vi "DriverStationSendData.vi"   [LabVIEW 2020]
doc: "This VI continously sends data from the robot to the FRC 4265 Dashboard, the joysticks, and the FIRST Driver Station. Data are only sent to the network tables when values change. Detailed sensor data are only sent when the user is currently viewing the Tune tab on the FRC 4265 Dashboard."
uses:
  <vilib>/Rock Robotics/WPI/DriverStation/WPI_DriverStationAllianceInfo.ctl
  0776bb0e-5b58-4af6-957d-bc8a00d122f2.vi
  c0b3d222-824d-4eea-b194-4551ccfede72.vi
  fb3b5982-3a93-47f1-af4b-9be2dbb142fb.vi
  9698e8dd-c256-4803-872d-8995bd52a814.vi
  549dd589-3d40-49fe-b500-ea8f2f2c089b.vi
  770be32f-1451-480f-be59-c95d907125ff.vi
  66123533-5387-4bde-a965-6a0533df74da.vi
  63beb643-7217-41a5-919e-8b0b42428238.vi
  f953088c-0ff5-4157-aadb-ae5236f80662.vi
  9b798e4d-9237-4864-9935-e997a6382231.vi
  bf36f1cc-a3b1-4189-9382-aff2debcdd91.vi
  09cab74e-98ba-4de8-92cd-b77291f0cae9.vi
  e0f98f21-d526-4ef5-b75c-6f3c78a33603.vi
  ae67384e-06ed-4288-bfa6-012d261b0193.vi
  36759aca-d9c6-44a3-918a-9a0e895c718f.vi
  d2dc3f3f-39b5-4c17-a933-05bbedc8d5d9.vi
  47e8091e-0604-4560-b6ee-932fcc40f94c.vi
  040c557e-2b24-4d13-8fef-d98c711cf45f.vi
  6883bb39-9618-44d1-87fc-0a8820399f5c.vi
  89115614-314f-44eb-b4c5-fafba5d31cd4.vi
  9f98788f-6f1b-4a83-a100-7d872b9f460c.vi
  d5b4d43d-cd94-4278-ad04-5030dc28ac17.vi
  f1b5b85a-7b65-4ee5-b0c1-040e47bf9d1e.vi
  126b0509-d7cb-49f5-b98e-abd766492b4e.vi
  120bb425-e072-480b-984e-eae4db04af5e.vi
  998fb6f4-27dd-4ee0-9bfc-5a2c9b2a219d.vi
  160f5f7d-3624-40a1-8964-721251a961b0.vi
  9695115c-43ac-455f-beff-ac1830b74b00.vi
  90b8ffb3-02b0-4f37-8578-c415475fcf1f.vi
  26471c2c-aca7-4047-a7cd-e40da11d04c1.vi
  0c9c2ce5-4f8f-4d2f-a61f-dde9fdddd21a.vi
  948ebb5e-1fee-45f5-b788-843df8d92f11.vi
  07cec073-88f4-4f05-94a3-d05e12405c4e.vi
  c10cd8a7-bdb7-4c92-ac5c-00af4ab7dc85.vi
  ce82ba1c-dcc2-498f-8d23-146b12230de2.vi
  cbbdf295-aa1d-4db8-8566-cac5820e4458.vi
  52d993e2-6fbc-4ee4-b085-b3f80a4c3067.vi
  5ccc8aa6-325d-4660-b060-52e30b1d582a.vi
  296afef1-bc02-48ee-92b6-09523bb21575.vi
  811948b9-57e2-4f47-a6f6-f2932d14082f.vi
  5739ca73-a30d-4c92-9c50-72d6edc45fc4.vi
  0620df73-5841-450f-a219-dd10bb38cbc0.vi
  fb087c59-fbb1-4979-ba7d-d29f083bcd8a.vi
  94826c24-d30e-4eee-b4d4-6d626a9b9fe7.vi
  fa7611ee-6daf-4341-84ec-bae2216748b8.vi
  8b25c428-5d86-4327-8799-14b0f475aaa3.vi
  26bfd72d-5ff1-456c-8357-2895bcab42df.vi
  12ad7fc7-8c22-4204-99a5-6d293ce0fad5.vi
  51dbaaa3-c108-440b-99ef-ee86c78a4638.vi
  6f39c387-5fba-42a0-a54d-01232661dc89.vi
  d8771982-752a-4faa-9266-2bef2163cf3a.vi
  a4ee2b99-23b1-4fe2-8107-6c56fb4f34ae.vi
  35ebf81f-d097-4745-a903-3018ca72664a.vi
  d6b922cd-d90c-4381-a0e2-4a950c41b267.vi
  cc938a22-4dac-4550-9998-d24c8aa0ec11.vi
  4a18f71a-ac32-4632-9b15-f0d0cf92b11d.vi
  7b6a1411-5027-49fa-871d-ec9f81e31f95.vi
  20dd8ad3-6bbc-4cac-b559-7f798e2b6680.vi
  5e95d400-1295-40c5-af46-ec5444c3a2ff.vi
  d5b53c9f-0752-48c4-83e9-94c6e20357af.vi
  a2a431f6-075f-4920-bddd-4a0a2690fbc3.vi
  63edfc8b-2713-4fb9-bbf0-712b13f7ed91.vi
  5dc304d7-e71b-4cd2-8d9d-954937278b50.vi
  2c1d3e71-7d83-4635-803e-5434fcaaade7.vi
  c227876e-c49d-4561-a8c1-0ac62d9f5df0.vi
  e617f737-58a4-4889-9924-01a8da667f92.vi
  a9076398-35a2-42a7-b542-3dd64d126b59.vi
  44842b00-b9c8-4b1f-a6e0-fc22f00ef89a.vi
  fb3b5982-3a93-47f1-af4b-9be2dbb142fb.vi/77c742ae-e671-49bb-a825-a6e8cebc9f63.vi
  9698e8dd-c256-4803-872d-8995bd52a814.vi/77c742ae-e671-49bb-a825-a6e8cebc9f63.vi
  549dd589-3d40-49fe-b500-ea8f2f2c089b.vi/77c742ae-e671-49bb-a825-a6e8cebc9f63.vi
  770be32f-1451-480f-be59-c95d907125ff.vi/77c742ae-e671-49bb-a825-a6e8cebc9f63.vi
  66123533-5387-4bde-a965-6a0533df74da.vi/77c742ae-e671-49bb-a825-a6e8cebc9f63.vi
  63beb643-7217-41a5-919e-8b0b42428238.vi/77c742ae-e671-49bb-a825-a6e8cebc9f63.vi
  f953088c-0ff5-4157-aadb-ae5236f80662.vi/77c742ae-e671-49bb-a825-a6e8cebc9f63.vi
  9b798e4d-9237-4864-9935-e997a6382231.vi/77c742ae-e671-49bb-a825-a6e8cebc9f63.vi
  bf36f1cc-a3b1-4189-9382-aff2debcdd91.vi/77c742ae-e671-49bb-a825-a6e8cebc9f63.vi
  09cab74e-98ba-4de8-92cd-b77291f0cae9.vi/77c742ae-e671-49bb-a825-a6e8cebc9f63.vi
  e0f98f21-d526-4ef5-b75c-6f3c78a33603.vi/77c742ae-e671-49bb-a825-a6e8cebc9f63.vi
  ae67384e-06ed-4288-bfa6-012d261b0193.vi/77c742ae-e671-49bb-a825-a6e8cebc9f63.vi
  36759aca-d9c6-44a3-918a-9a0e895c718f.vi/77c742ae-e671-49bb-a825-a6e8cebc9f63.vi
  d2dc3f3f-39b5-4c17-a933-05bbedc8d5d9.vi/77c742ae-e671-49bb-a825-a6e8cebc9f63.vi
  47e8091e-0604-4560-b6ee-932fcc40f94c.vi/77c742ae-e671-49bb-a825-a6e8cebc9f63.vi
  040c557e-2b24-4d13-8fef-d98c711cf45f.vi/77c742ae-e671-49bb-a825-a6e8cebc9f63.vi
  6883bb39-9618-44d1-87fc-0a8820399f5c.vi/77c742ae-e671-49bb-a825-a6e8cebc9f63.vi
  89115614-314f-44eb-b4c5-fafba5d31cd4.vi/77c742ae-e671-49bb-a825-a6e8cebc9f63.vi
  9f98788f-6f1b-4a83-a100-7d872b9f460c.vi/77c742ae-e671-49bb-a825-a6e8cebc9f63.vi
  d5b4d43d-cd94-4278-ad04-5030dc28ac17.vi/77c742ae-e671-49bb-a825-a6e8cebc9f63.vi
  f1b5b85a-7b65-4ee5-b0c1-040e47bf9d1e.vi/77c742ae-e671-49bb-a825-a6e8cebc9f63.vi
  126b0509-d7cb-49f5-b98e-abd766492b4e.vi/77c742ae-e671-49bb-a825-a6e8cebc9f63.vi
  120bb425-e072-480b-984e-eae4db04af5e.vi/77c742ae-e671-49bb-a825-a6e8cebc9f63.vi
  998fb6f4-27dd-4ee0-9bfc-5a2c9b2a219d.vi/77c742ae-e671-49bb-a825-a6e8cebc9f63.vi
  160f5f7d-3624-40a1-8964-721251a961b0.vi/77c742ae-e671-49bb-a825-a6e8cebc9f63.vi
  9695115c-43ac-455f-beff-ac1830b74b00.vi/77c742ae-e671-49bb-a825-a6e8cebc9f63.vi
  90b8ffb3-02b0-4f37-8578-c415475fcf1f.vi/77c742ae-e671-49bb-a825-a6e8cebc9f63.vi
  26471c2c-aca7-4047-a7cd-e40da11d04c1.vi/77c742ae-e671-49bb-a825-a6e8cebc9f63.vi
  0c9c2ce5-4f8f-4d2f-a61f-dde9fdddd21a.vi/77c742ae-e671-49bb-a825-a6e8cebc9f63.vi
  948ebb5e-1fee-45f5-b788-843df8d92f11.vi/77c742ae-e671-49bb-a825-a6e8cebc9f63.vi
  07cec073-88f4-4f05-94a3-d05e12405c4e.vi/77c742ae-e671-49bb-a825-a6e8cebc9f63.vi
  c10cd8a7-bdb7-4c92-ac5c-00af4ab7dc85.vi/77c742ae-e671-49bb-a825-a6e8cebc9f63.vi
  ce82ba1c-dcc2-498f-8d23-146b12230de2.vi/77c742ae-e671-49bb-a825-a6e8cebc9f63.vi
  cbbdf295-aa1d-4db8-8566-cac5820e4458.vi/77c742ae-e671-49bb-a825-a6e8cebc9f63.vi
  52d993e2-6fbc-4ee4-b085-b3f80a4c3067.vi/77c742ae-e671-49bb-a825-a6e8cebc9f63.vi
  5ccc8aa6-325d-4660-b060-52e30b1d582a.vi/77c742ae-e671-49bb-a825-a6e8cebc9f63.vi
  296afef1-bc02-48ee-92b6-09523bb21575.vi/77c742ae-e671-49bb-a825-a6e8cebc9f63.vi
  811948b9-57e2-4f47-a6f6-f2932d14082f.vi/77c742ae-e671-49bb-a825-a6e8cebc9f63.vi
  5739ca73-a30d-4c92-9c50-72d6edc45fc4.vi/77c742ae-e671-49bb-a825-a6e8cebc9f63.vi
  0620df73-5841-450f-a219-dd10bb38cbc0.vi/77c742ae-e671-49bb-a825-a6e8cebc9f63.vi
  fb087c59-fbb1-4979-ba7d-d29f083bcd8a.vi/77c742ae-e671-49bb-a825-a6e8cebc9f63.vi
  94826c24-d30e-4eee-b4d4-6d626a9b9fe7.vi/77c742ae-e671-49bb-a825-a6e8cebc9f63.vi
  fa7611ee-6daf-4341-84ec-bae2216748b8.vi/77c742ae-e671-49bb-a825-a6e8cebc9f63.vi
  8b25c428-5d86-4327-8799-14b0f475aaa3.vi/77c742ae-e671-49bb-a825-a6e8cebc9f63.vi
  26bfd72d-5ff1-456c-8357-2895bcab42df.vi/77c742ae-e671-49bb-a825-a6e8cebc9f63.vi
  12ad7fc7-8c22-4204-99a5-6d293ce0fad5.vi/77c742ae-e671-49bb-a825-a6e8cebc9f63.vi
  51dbaaa3-c108-440b-99ef-ee86c78a4638.vi/77c742ae-e671-49bb-a825-a6e8cebc9f63.vi
  6f39c387-5fba-42a0-a54d-01232661dc89.vi/77c742ae-e671-49bb-a825-a6e8cebc9f63.vi
  d8771982-752a-4faa-9266-2bef2163cf3a.vi/77c742ae-e671-49bb-a825-a6e8cebc9f63.vi
  a4ee2b99-23b1-4fe2-8107-6c56fb4f34ae.vi/77c742ae-e671-49bb-a825-a6e8cebc9f63.vi
  35ebf81f-d097-4745-a903-3018ca72664a.vi/77c742ae-e671-49bb-a825-a6e8cebc9f63.vi
  d6b922cd-d90c-4381-a0e2-4a950c41b267.vi/77c742ae-e671-49bb-a825-a6e8cebc9f63.vi
  cc938a22-4dac-4550-9998-d24c8aa0ec11.vi/77c742ae-e671-49bb-a825-a6e8cebc9f63.vi
  4a18f71a-ac32-4632-9b15-f0d0cf92b11d.vi/77c742ae-e671-49bb-a825-a6e8cebc9f63.vi
  7b6a1411-5027-49fa-871d-ec9f81e31f95.vi/77c742ae-e671-49bb-a825-a6e8cebc9f63.vi
  20dd8ad3-6bbc-4cac-b559-7f798e2b6680.vi/77c742ae-e671-49bb-a825-a6e8cebc9f63.vi
  5e95d400-1295-40c5-af46-ec5444c3a2ff.vi/77c742ae-e671-49bb-a825-a6e8cebc9f63.vi
  d5b53c9f-0752-48c4-83e9-94c6e20357af.vi/77c742ae-e671-49bb-a825-a6e8cebc9f63.vi
  a2a431f6-075f-4920-bddd-4a0a2690fbc3.vi/77c742ae-e671-49bb-a825-a6e8cebc9f63.vi
  63edfc8b-2713-4fb9-bbf0-712b13f7ed91.vi/77c742ae-e671-49bb-a825-a6e8cebc9f63.vi
  5dc304d7-e71b-4cd2-8d9d-954937278b50.vi/77c742ae-e671-49bb-a825-a6e8cebc9f63.vi
  2c1d3e71-7d83-4635-803e-5434fcaaade7.vi/77c742ae-e671-49bb-a825-a6e8cebc9f63.vi
  c227876e-c49d-4561-a8c1-0ac62d9f5df0.vi/77c742ae-e671-49bb-a825-a6e8cebc9f63.vi
  e617f737-58a4-4889-9924-01a8da667f92.vi/77c742ae-e671-49bb-a825-a6e8cebc9f63.vi
  a9076398-35a2-42a7-b542-3dd64d126b59.vi/77c742ae-e671-49bb-a825-a6e8cebc9f63.vi
  44842b00-b9c8-4b1f-a6e0-fc22f00ef89a.vi/77c742ae-e671-49bb-a825-a6e8cebc9f63.vi
  GlobalDriverStationData.vi
  GlobalAutonomous.vi
  <vilib>/Rock Robotics/Network Tables/NT Write String Array.vi
  GlobalDrivebase.vi
  <vilib>/Rock Robotics/Network Tables/NT Write Number.vi
  GlobalMiscellaneous.vi
  <vilib>/Rock Robotics/Network Tables/NT Write String.vi
  GlobalPoseAndTargeting.vi
  GlobalArm.vi
  <vilib>/Rock Robotics/Network Tables/NT Write Numeric Array.vi
  Timer.vi
  <vilib>/Rock Robotics/Network Tables/NT Write Boolean Array.vi
  GlobalGripper.vi
  <vilib>/Rock Robotics/Network Tables/NT Write Float Array.vi
  <vilib>/Rock Robotics/Network Tables/NT Write Boolean.vi
  95d3f975-1fa3-4bf8-b07d-de262660b4dc.vi
  <vilib>/Rock Robotics/Network Tables/NT Write Variant.vi
types:
  T1 = typedef "WPI_DriverStationAllianceInfo.ctl" = enum16{"Red", "Blue", "Invalid"}
  T2 = cluster{"X(in)":dbl, "Y(in)":dbl, "Count":i32, "Timestamp(ms)":u32, "Piece":enum16{"Cube", "Cone"}}[]
  T3 = cluster{"X(in)":bool, "Y(in)":bool, "Count":bool, "Timestamp(ms)":bool, "Piece":bool}[]
  T4 = enum16{"Low Gear", "High Gear", "Transiting", "Unknown", "Force Low Gear"}
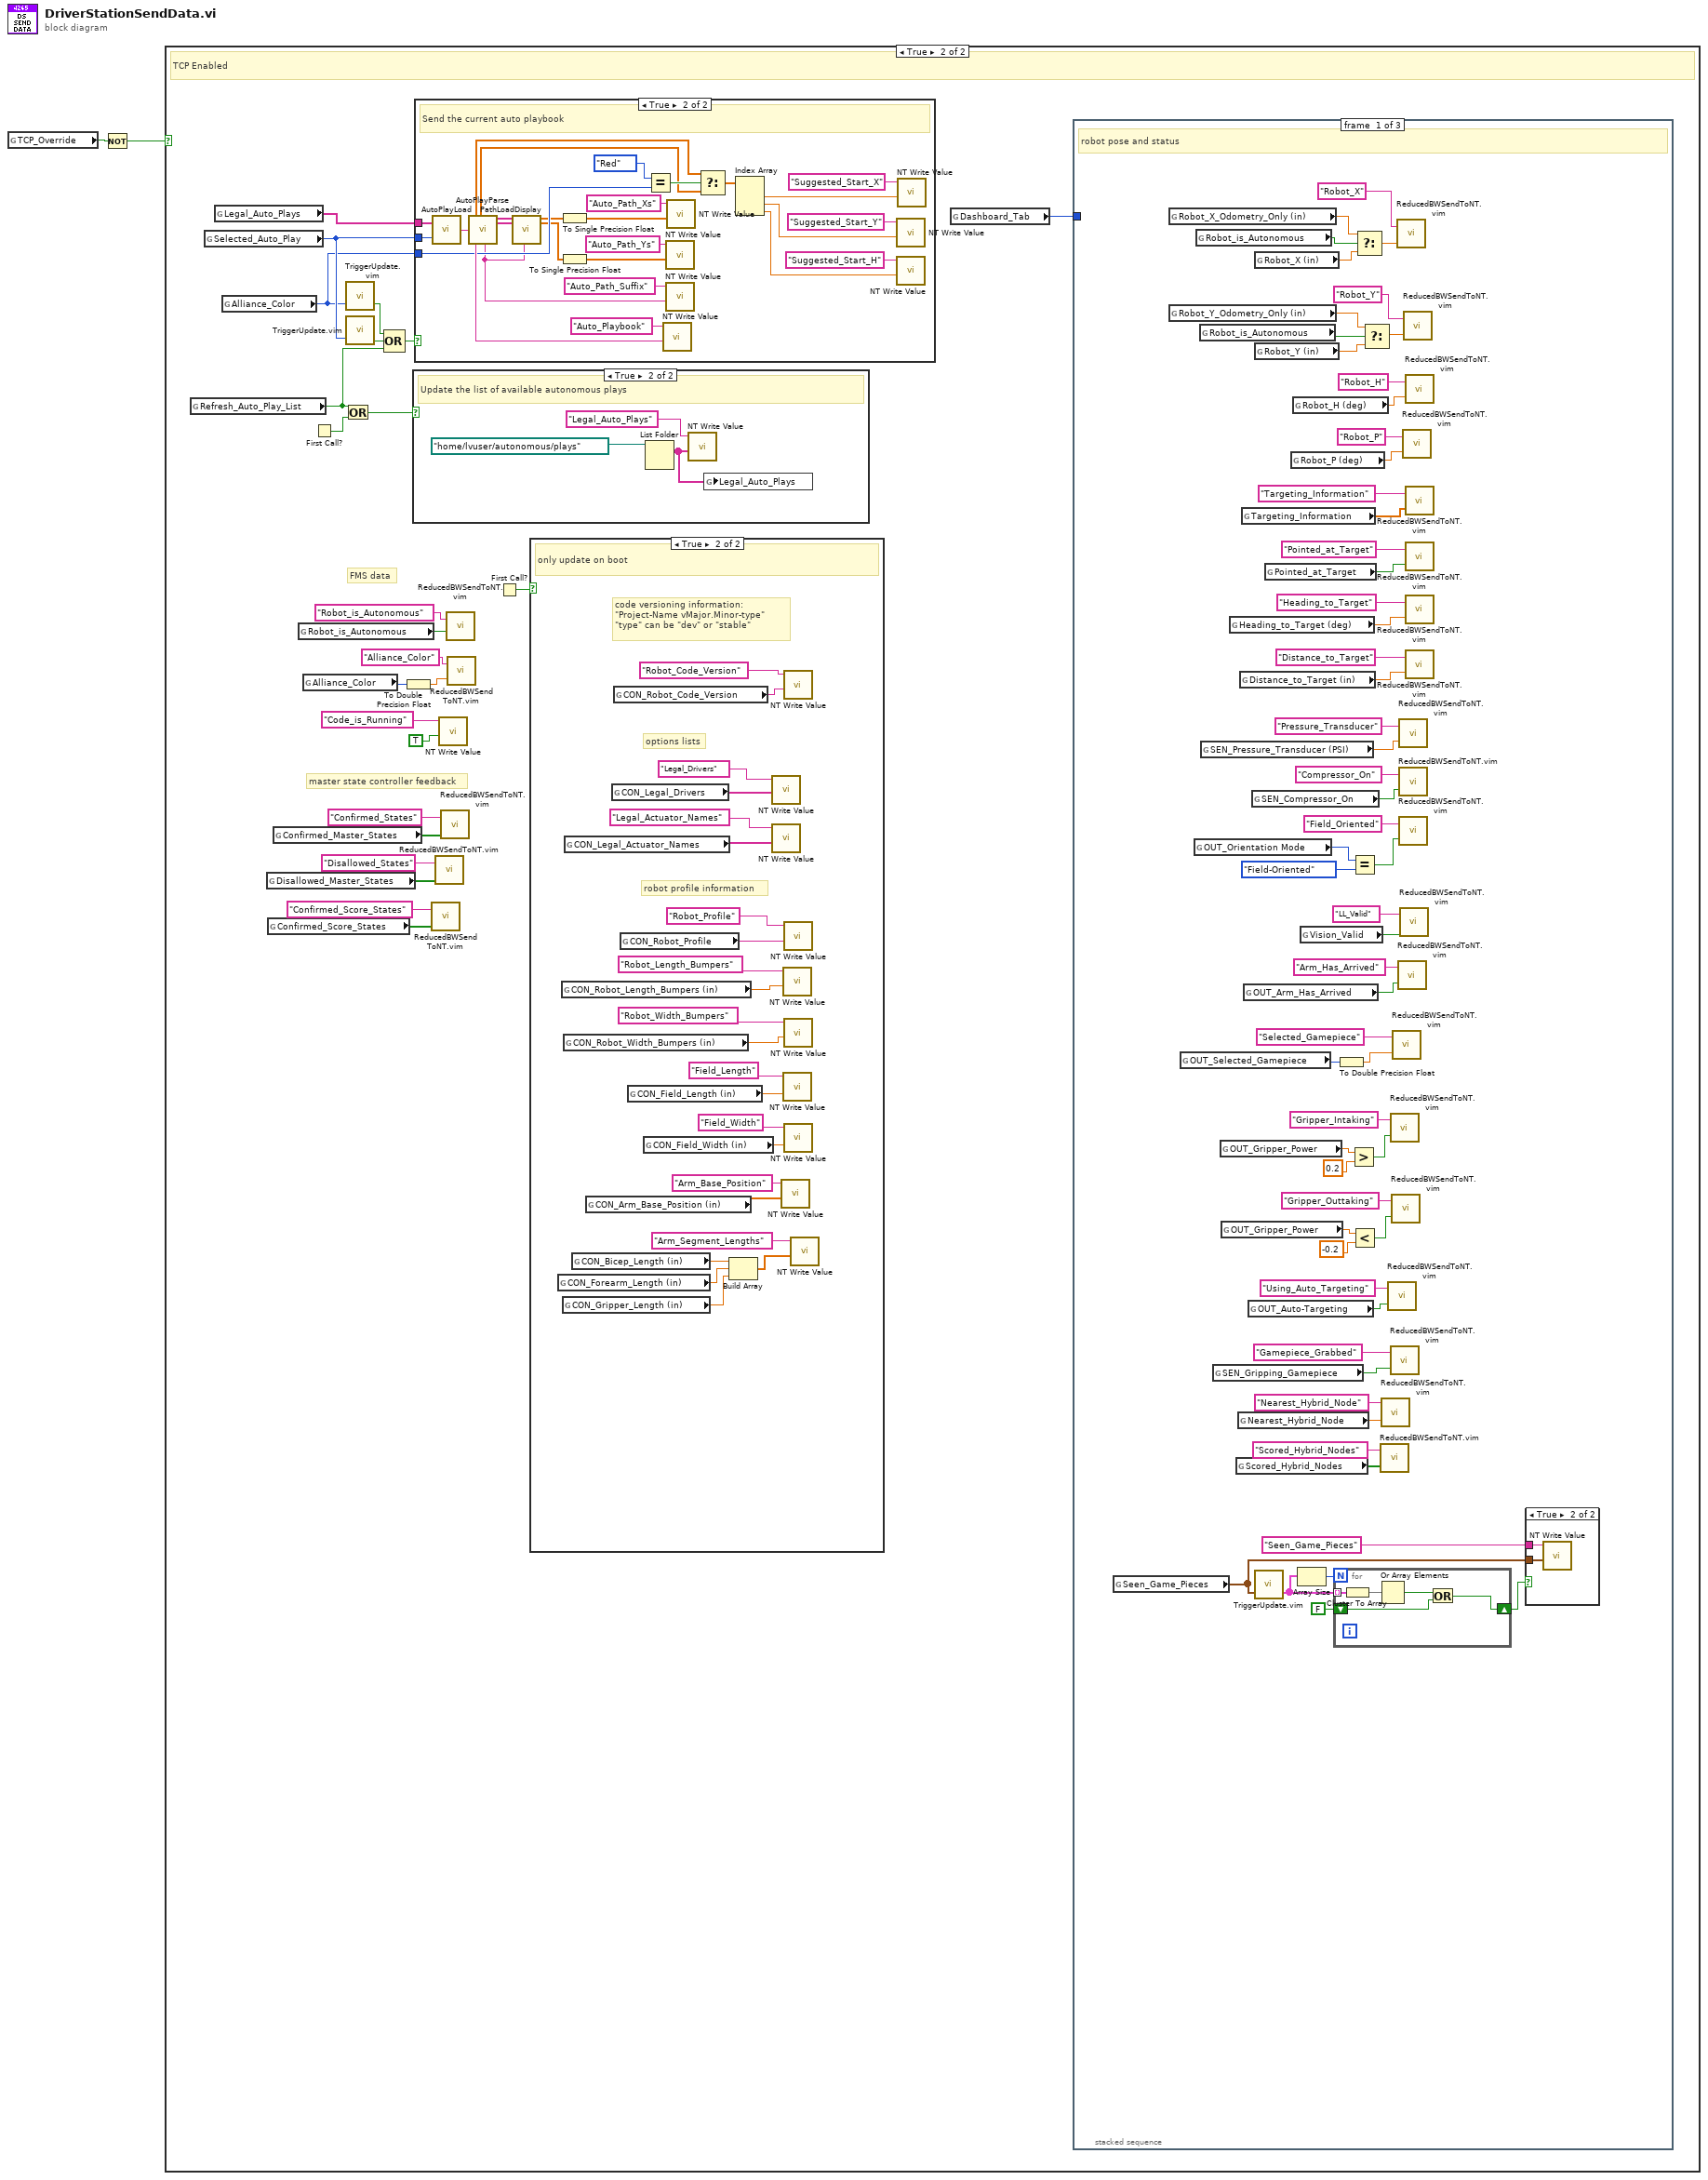
[diagram p0: block diagram]
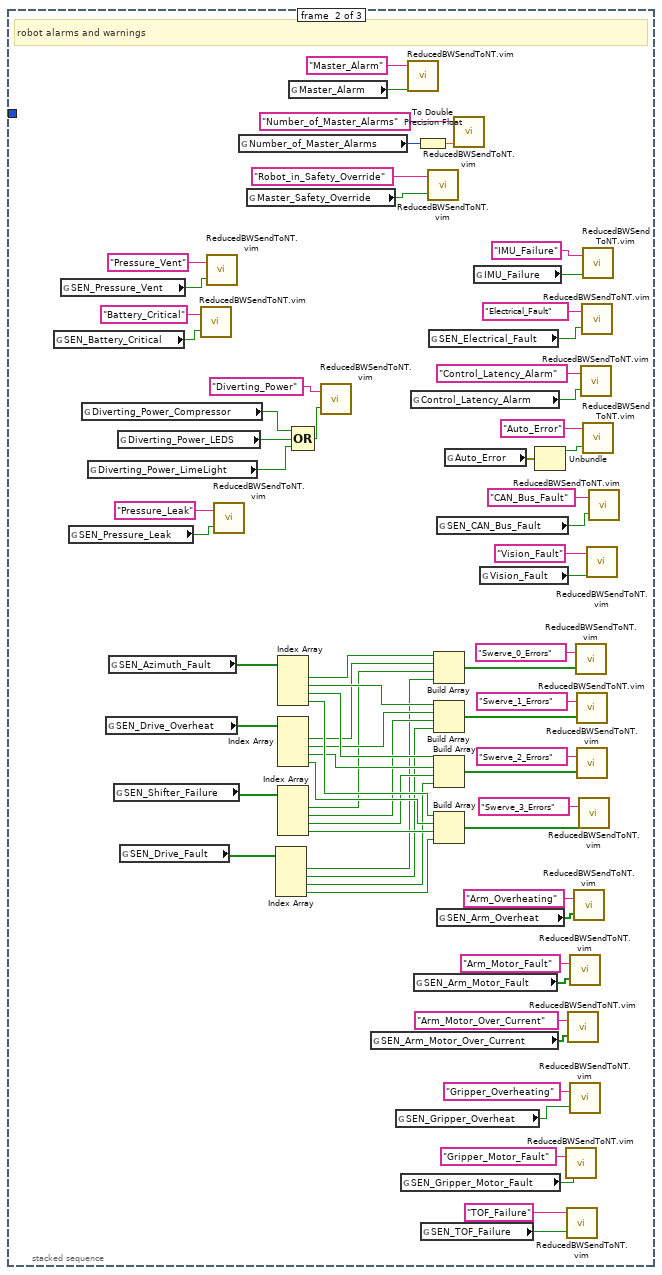
[diagram p4: hidden frame]
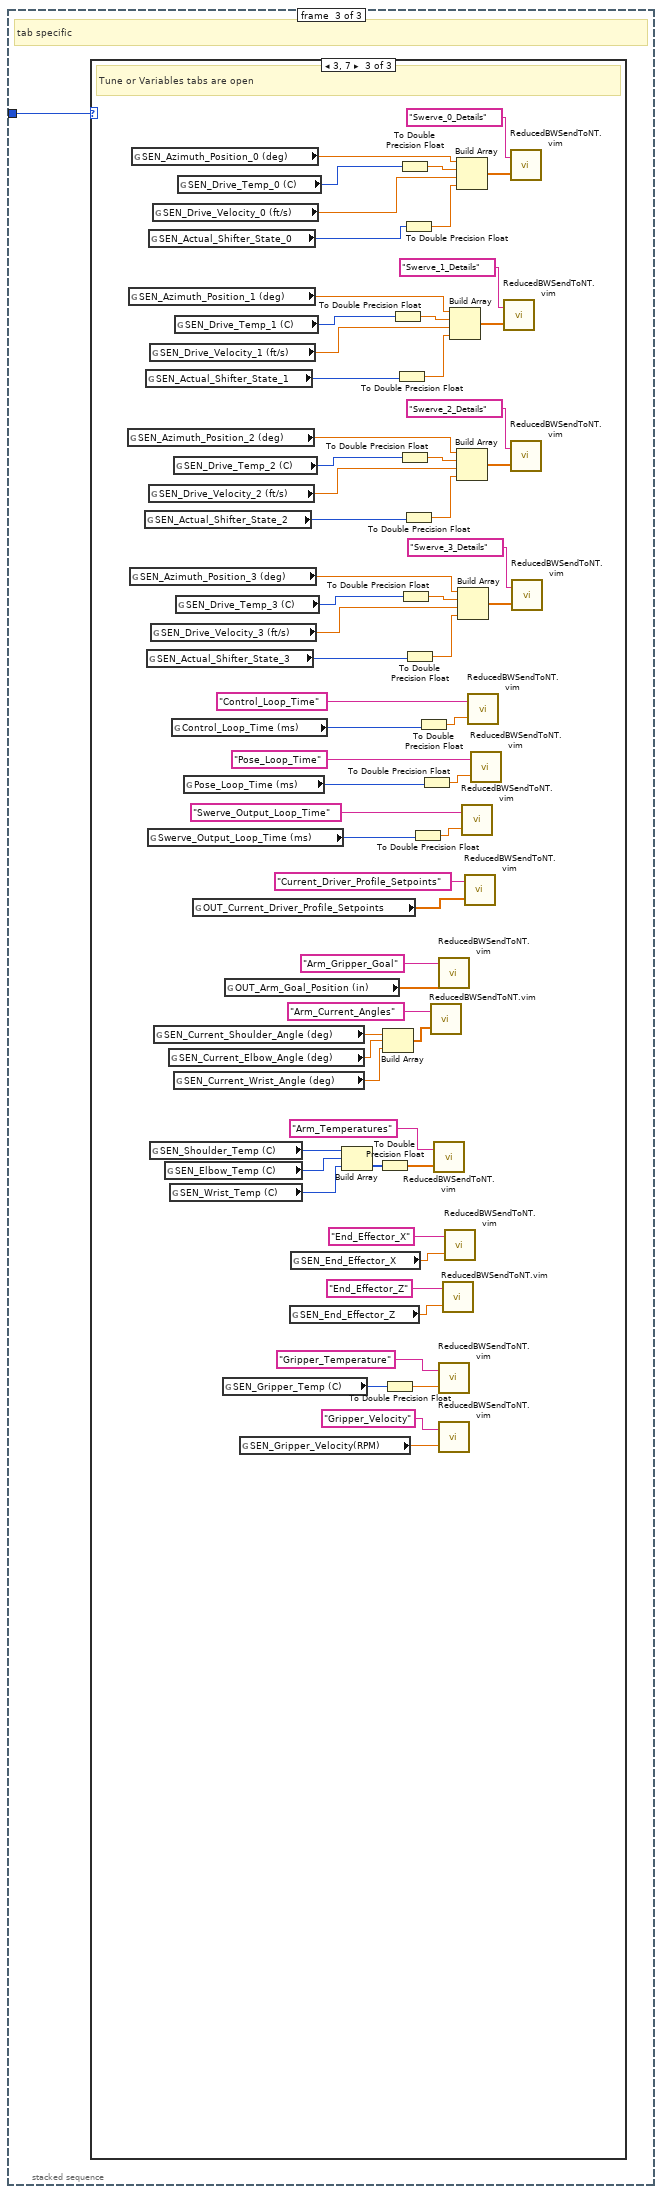
[diagram p5: hidden frame]
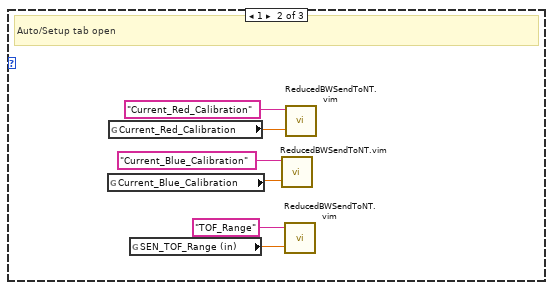
[diagram p7: hidden frame]
diagram:
  n1 = global read "GlobalDriverStationData.vi" "TCP_Override"() -> (w2:bool)
  n2 = Not(x=w2) -> (.not. x?=w1:bool)
  n3 = case shown="True" w1 {
    frame False {
      # "TCP Disabled"
    }
    frame True {
      # "FMS data"
      # "master state controller feedback"
      # "TCP Enabled"
      n4 = global read "GlobalDriverStationData.vi" "Refresh_Auto_Play_List"() -> (w22:bool)
      n5 = global read "GlobalDriverStationData.vi" "Selected_Auto_Play"() -> (w9:u16)
      n6 = global read "GlobalAutonomous.vi" "Legal_Auto_Plays"() -> (w10:string[])
      n7 = global read "GlobalDriverStationData.vi" "Alliance_Color"() -> (w7:T1)
      n8 = global read "GlobalMiscellaneous.vi" "Disallowed_Master_States"() -> (w12:bool[])
      n9 = global read "GlobalArm.vi" "Confirmed_Score_States"() -> (w5:bool[])
      n10 = global read "GlobalMiscellaneous.vi" "Confirmed_Master_States"() -> (w14:bool[])
      n11 = global read "GlobalDriverStationData.vi" "Robot_is_Autonomous"() -> (w18:bool)
      n12 = global read "GlobalDriverStationData.vi" "Alliance_Color"() -> (w20:T1)
      n13 = First Call?() -> (First Call?: T/F=w26:bool)
      n14 = Or(x=w22, y=w26) -> (x .or. y?=w25:bool)
      n15 = call "TriggerUpdate.vim"("Trigger"=w7) -> ("Update"=w8:bool)  [unwired: 2 in]
      n16 = call "TriggerUpdate.vim"("Trigger"=w9) -> ("Update"=w24:bool)  [unwired: 2 in]
      n17 = Compound Arithmetic op=OR(w8, w24, w22) -> (w23:bool)
      n18 = To Double Precision Float(number=w20) -> (double precision float=w16:dbl)
      n19 = case shown="True" w25 {
        frame False {
        }
        frame True {
          # "Update the list of available autonomous plays"
          n20 = List Folder(path=path "/home/lvuser/autonomous/plays") -> (filenames=w286:string[])  [unwired: 3 in, 3 out]
          n21 = call-poly <vilib>:"NT Write Value.vi"("value"=w286, "name"="Legal_Auto_Plays" ("Name")) -> ()  [unwired: 9 in, 1 out]
          n22 = global write "GlobalAutonomous.vi" "Legal_Auto_Plays"(w286) -> ()
        }
      }
      n23 = case shown="True" w23 {
        tunnel: w9 -> [_ w283]
        tunnel: w10 -> [_ w282]
        tunnel: w7 -> [_ w278]
        frame False {
        }
        frame True {
          # "Send the current auto playbook"
          n24 = call "AutoPlayLoad.vi"("Selected Auto Play"=w283, "Available Auto Plays"=w282) -> ("Loaded Auto Play"=w284:string)
          n25 = call "AutoPlayParse.vi"("Loaded Auto Play"=w284) -> ("Suggested Start Red"=w276:dbl[], "Full Auto Play Text"=w281:string, "Suggested Start Blue"=w275:dbl[], "Autonomous Path Suffix"=w265:string, "Drive Command Strings"=w267:string[], "Drive Parameter Strings"=w266:string[])  [unwired: 10 in, 3 out]
          n26 = call "PathLoadDisplay.vi"("Drive Command Strings"=w267, "Drive Parameter Strings"=w266, "Autonomous Path Suffix"=w265) -> ("Path X Coordinates (in)"=w263:dbl[], "Path Y Coordinates (in)"=w261:dbl[])  [unwired: 15 in]
          n27 = To Single Precision Float(number=w263) -> (single precision float=w260:sgl[])
          n28 = To Single Precision Float(number=w261) -> (single precision float=w259:sgl[])
          n29 = Equal?(x=WPI_DriverStationAllianceInfo."Red", y=w278) -> (x = y?=w279:bool)
          n30 = call-poly <vilib>:"NT Write Value.vi"("value"=w281, "name"="Auto_Playbook" ("Name")) -> ()  [unwired: 9 in, 1 out]
          n31 = call-poly <vilib>:"NT Write Value.vi"("value"=w259, "name"="Auto_Path_Ys" ("Name")) -> ()  [unwired: 9 in, 1 out]
          n32 = call-poly <vilib>:"NT Write Value.vi"("value"=w265, "name"="Auto_Path_Suffix" ("Name")) -> ()  [unwired: 9 in, 1 out]
          n33 = call-poly <vilib>:"NT Write Value.vi"("value"=w260, "name"="Auto_Path_Xs" ("Name")) -> ()  [unwired: 9 in, 1 out]
          n34 = Select(t=w276, s=w279, f=w275) -> (s? t:f=w274:dbl[])
          n35 = Index Array(array=w274) -> (element #1=w270:dbl, element #2=w269:dbl, element #3=w268:dbl)  [unwired: 3 in]
          n36 = call-poly <vilib>:"NT Write Value.vi"("value"=w269, "name"="Suggested_Start_Y" ("Name")) -> ()  [unwired: 9 in, 1 out]
          n37 = call-poly <vilib>:"NT Write Value.vi"("value"=w268, "name"="Suggested_Start_H" ("Name")) -> ()  [unwired: 9 in, 1 out]
          n38 = call-poly <vilib>:"NT Write Value.vi"("value"=w270, "name"="Suggested_Start_X" ("Name")) -> ()  [unwired: 9 in, 1 out]
        }
      }
      n39 = call "ReducedBWSendToNT.vim"("Value In"=w5, "NT Name"="Confirmed_Score_States" ("Name")) -> ()  [unwired: 1 out]
      n40 = call "ReducedBWSendToNT.vim"("Value In"=w12, "NT Name"="Disallowed_States" ("Name")) -> ()  [unwired: 1 out]
      n41 = call-poly <vilib>:"NT Write Value.vi"("value"=TRUE, "name"="Code_is_Running" ("NT Name")) -> ()  [unwired: 9 in, 1 out]
      n42 = call "ReducedBWSendToNT.vim"("Value In"=w14, "NT Name"="Confirmed_States" ("Name")) -> ()  [unwired: 1 out]
      n43 = call "ReducedBWSendToNT.vim"("Value In"=w18, "NT Name"="Robot_is_Autonomous") -> ()  [unwired: 1 out]
      n44 = call "ReducedBWSendToNT.vim"("Value In"=w16, "NT Name"="Alliance_Color") -> ()  [unwired: 1 out]
      n45 = First Call?() -> (First Call?: T/F=w21:bool)
      n46 = case shown="True" w21 {
        frame False {
        }
        frame True {
          # "robot profile information"
          # "options lists"
          # "code versioning information:\n\"Project-Name vMajor.Minor-type\"\n\"type\" can be \"dev\" or \"stable\""
          # "only update on boot"
          n47 = global read "GlobalArm.vi" "CON_Forearm_Length (in)"() -> (w238:dbl)
          n48 = global read "GlobalDrivebase.vi" "CON_Robot_Length_Bumpers (in)"() -> (w252:dbl)
          n49 = global read "GlobalArm.vi" "CON_Gripper_Length (in)"() -> (w237:dbl)
          n50 = global read "GlobalDrivebase.vi" "CON_Robot_Width_Bumpers (in)"() -> (w251:dbl)
          n51 = global read "GlobalMiscellaneous.vi" "CON_Legal_Actuator_Names"() -> (w249:string[])
          n52 = global read "GlobalArm.vi" "CON_Bicep_Length (in)"() -> (w239:dbl)
          n53 = global read "GlobalArm.vi" "CON_Arm_Base_Position (in)"() -> (w241:dbl[])
          n54 = global read "GlobalDrivebase.vi" "CON_Legal_Drivers"() -> (w250:string[])
          n55 = global read "GlobalMiscellaneous.vi" "CON_Robot_Code_Version"() -> (w247:string)
          n56 = global read "GlobalMiscellaneous.vi" "CON_Robot_Profile"() -> (w248:string)
          n57 = global read "GlobalPoseAndTargeting.vi" "CON_Field_Length (in)"() -> (w246:dbl)
          n58 = global read "GlobalPoseAndTargeting.vi" "CON_Field_Width (in)"() -> (w243:dbl)
          n59 = Build Array(w239, w238, w237) -> (w236:dbl[])
          n60 = call-poly <vilib>:"NT Write Value.vi"("value"=w250, "name"="Legal_Drivers" ("Name")) -> ()  [unwired: 9 in, 1 out]
          n61 = call-poly <vilib>:"NT Write Value.vi"("value"=w249, "name"="Legal_Actuator_Names" ("Name")) -> ()  [unwired: 9 in, 1 out]
          n62 = call-poly <vilib>:"NT Write Value.vi"("value"=w241, "name"="Arm_Base_Position") -> ()  [unwired: 9 in, 1 out]
          n63 = call-poly <vilib>:"NT Write Value.vi"("value"=w252, "name"="Robot_Length_Bumpers" ("Name")) -> ()  [unwired: 9 in, 1 out]
          n64 = call-poly <vilib>:"NT Write Value.vi"("value"=w246, "name"="Field_Length" ("Name")) -> ()  [unwired: 9 in, 1 out]
          n65 = call-poly <vilib>:"NT Write Value.vi"("value"=w247, "name"="Robot_Code_Version" ("Name")) -> ()  [unwired: 9 in, 1 out]
          n66 = call-poly <vilib>:"NT Write Value.vi"("value"=w248, "name"="Robot_Profile" ("Name")) -> ()  [unwired: 9 in, 1 out]
          n67 = call-poly <vilib>:"NT Write Value.vi"("value"=w251, "name"="Robot_Width_Bumpers" ("Name")) -> ()  [unwired: 9 in, 1 out]
          n68 = call-poly <vilib>:"NT Write Value.vi"("value"=w243, "name"="Field_Width" ("Name")) -> ()  [unwired: 9 in, 1 out]
          n69 = call-poly <vilib>:"NT Write Value.vi"("value"=w236, "name"="Arm_Segment_Lengths") -> ()  [unwired: 9 in, 1 out]
        }
      }
      n70 = global read "GlobalDriverStationData.vi" "Dashboard_Tab"() -> (w11:i8)
      n71 = stacked-sequence {
        tunnel: w11 -> [_ _ w164]
        frame #0 {
          # "robot pose and status"
          n72 = global read "GlobalPoseAndTargeting.vi" "Seen_Game_Pieces"() -> (w31:T2)
          n73 = global read "GlobalPoseAndTargeting.vi" "Robot_X_Odometry_Only (in)"() -> (w80:dbl)
          n74 = global read "GlobalPoseAndTargeting.vi" "Robot_Y_Odometry_Only (in)"() -> (w81:dbl)
          n75 = global read "GlobalArm.vi" "OUT_Selected_Gamepiece"() -> (w50:enum16{"Cube", "Cone"})
          n76 = global read "GlobalDrivebase.vi" "OUT_Orientation Mode"() -> (w64:enum16{"Robot-Oriented", "Field-Oriented"})
          n77 = global read "GlobalDriverStationData.vi" "Robot_is_Autonomous"() -> (w84:bool)
          n78 = global read "GlobalDriverStationData.vi" "Robot_is_Autonomous"() -> (w85:bool)
          n79 = global read "GlobalMiscellaneous.vi" "SEN_Pressure_Transducer (PSI)"() -> (w63:dbl)
          n80 = global read "GlobalGripper.vi" "SEN_Gripping_Gamepiece"() -> (w37:bool)
          n81 = global read "GlobalGripper.vi" "OUT_Gripper_Power"() -> (w47:dbl)
          n82 = global read "GlobalGripper.vi" "OUT_Gripper_Power"() -> (w43:dbl)
          n83 = global read "GlobalPoseAndTargeting.vi" "Heading_to_Target (deg)"() -> (w55:dbl)
          n84 = global read "GlobalPoseAndTargeting.vi" "Scored_Hybrid_Nodes"() -> (w34:bool[])
          n85 = global read "GlobalPoseAndTargeting.vi" "Nearest_Hybrid_Node"() -> (w36:dbl)
          n86 = global read "GlobalPoseAndTargeting.vi" "Distance_to_Target (in)"() -> (w53:dbl)
          n87 = global read "GlobalPoseAndTargeting.vi" "Targeting_Information"() -> (w76:dbl[])
          n88 = global read "GlobalArm.vi" "OUT_Arm_Has_Arrived"() -> (w60:bool)
          n89 = global read "GlobalDrivebase.vi" "OUT_Auto-Targeting"() -> (w39:bool)
          n90 = global read "GlobalMiscellaneous.vi" "SEN_Compressor_On"() -> (w62:bool)
          n91 = global read "GlobalPoseAndTargeting.vi" "Robot_X (in)"() -> (w78:dbl)
          n92 = global read "GlobalPoseAndTargeting.vi" "Robot_Y (in)"() -> (w79:dbl)
          n93 = call "TriggerUpdate.vim"("Trigger"=w31) -> ("Update"=w29:T3)  [unwired: 2 in]
          n94 = global read "GlobalPoseAndTargeting.vi" "Pointed_at_Target"() -> (w57:bool)
          n95 = global read "GlobalPoseAndTargeting.vi" "Robot_P (deg)"() -> (w59:dbl)
          n96 = global read "GlobalPoseAndTargeting.vi" "Robot_H (deg)"() -> (w77:dbl)
          n97 = Array Size(array=w29) -> (size(s)=w30:i32)
          n98 = global read "GlobalPoseAndTargeting.vi" "Vision_Valid"() -> (w70:bool)
          n99 = for {
            N: w30 -> [_]
            tunnel: w29 -> [w90] mode=indexing
            shift-right: [w86] -> w27
            shift-left: FALSE -> [w87]
            n100 = Cluster To Array(cluster=w90) -> (array=w89:bool[])
            n101 = Or Array Elements(Boolean array=w89) -> (logical OR=w88:bool)
            n102 = Or(x=w88, y=w87) -> (x .or. y?=w86:bool)
          }
          n103 = To Double Precision Float(number=w50) -> (double precision float=w49:dbl)
          n104 = Greater?(x=w47, y=0.2) -> (0:w45:bool)
          n105 = Equal?(x=w64, y=enum16{"Robot-Oriented", "Field-Oriented"}."Field-Oriented") -> (x = y?=w71:bool)
          n106 = Less?(x=w43, y=-0.2) -> (x < y?=w41:bool)
          n107 = Select(t=w80, s=w84, f=w78) -> (s? t:f=w82:dbl)
          n108 = Select(t=w81, s=w85, f=w79) -> (s? t:f=w83:dbl)
          n109 = call "ReducedBWSendToNT.vim"("Value In"=w34, "NT Name"="Scored_Hybrid_Nodes") -> ()  [unwired: 1 out]
          n110 = call "ReducedBWSendToNT.vim"("Value In"=w36, "NT Name"="Nearest_Hybrid_Node") -> ()  [unwired: 1 out]
          n111 = call "ReducedBWSendToNT.vim"("Value In"=w39, "NT Name"="Using_Auto_Targeting" ("Name")) -> ()  [unwired: 1 out]
          n112 = call "ReducedBWSendToNT.vim"("Value In"=w45, "NT Name"="Gripper_Intaking" ("Name")) -> ()  [unwired: 1 out]
          n113 = call "ReducedBWSendToNT.vim"("Value In"=w37, "NT Name"="Gamepiece_Grabbed" ("Name")) -> ()  [unwired: 1 out]
          n114 = call "ReducedBWSendToNT.vim"("Value In"=w41, "NT Name"="Gripper_Outtaking" ("Name")) -> ()  [unwired: 1 out]
          n115 = call "ReducedBWSendToNT.vim"("Value In"=w49, "NT Name"="Selected_Gamepiece" ("Name")) -> ()  [unwired: 1 out]
          n116 = call "ReducedBWSendToNT.vim"("Value In"=w82, "NT Name"="Robot_X" ("Name")) -> ()  [unwired: 1 out]
          n117 = call "ReducedBWSendToNT.vim"("Value In"=w60, "NT Name"="Arm_Has_Arrived" ("Name")) -> ()  [unwired: 1 out]
          n118 = call "ReducedBWSendToNT.vim"("Value In"=w63, "NT Name"="Pressure_Transducer" ("Name")) -> ()  [unwired: 1 out]
          n119 = call "ReducedBWSendToNT.vim"("Value In"=w62, "NT Name"="Compressor_On" ("Name")) -> ()  [unwired: 1 out]
          n120 = call "ReducedBWSendToNT.vim"("Value In"=w71, "NT Name"="Field_Oriented" ("Name")) -> ()  [unwired: 1 out]
          n121 = call "ReducedBWSendToNT.vim"("Value In"=w70, "NT Name"="LL_Valid" ("Name")) -> ()  [unwired: 1 out]
          n122 = call "ReducedBWSendToNT.vim"("Value In"=w59, "NT Name"="Robot_P" ("Name")) -> ()  [unwired: 1 out]
          n123 = call "ReducedBWSendToNT.vim"("Value In"=w83, "NT Name"="Robot_Y" ("Name")) -> ()  [unwired: 1 out]
          n124 = call "ReducedBWSendToNT.vim"("Value In"=w77, "NT Name"="Robot_H" ("Name")) -> ()  [unwired: 1 out]
          n125 = call "ReducedBWSendToNT.vim"("Value In"=w76, "NT Name"="Targeting_Information" ("Name")) -> ()  [unwired: 1 out]
          n126 = call "ReducedBWSendToNT.vim"("Value In"=w57, "NT Name"="Pointed_at_Target" ("Name")) -> ()  [unwired: 1 out]
          n127 = call "ReducedBWSendToNT.vim"("Value In"=w55, "NT Name"="Heading_to_Target" ("Name")) -> ()  [unwired: 1 out]
          n128 = call "ReducedBWSendToNT.vim"("Value In"=w53, "NT Name"="Distance_to_Target" ("Name")) -> ()  [unwired: 1 out]
          n129 = case shown="True" w27 {
            tunnel: w31 -> [_ w91]
            tunnel: "Seen_Game_Pieces" ("NT Name") -> [_ w92]
            frame False {
            }
            frame True {
              n130 = call-poly <vilib>:"NT Write Value.vi"("variant"=w91, "name"=w92) -> ()  [unwired: 9 in, 1 out]
            }
          }
        }
        frame #1 {
          # "robot alarms and warnings"
          n131 = global read "GlobalMiscellaneous.vi" "SEN_Battery_Critical"() -> (w114:bool)
          n132 = global read "GlobalMiscellaneous.vi" "SEN_Pressure_Vent"() -> (w115:bool)
          n133 = global read "GlobalMiscellaneous.vi" "SEN_Pressure_Leak"() -> (w111:bool)
          n134 = global read "GlobalMiscellaneous.vi" "Diverting_Power_Compressor"() -> (w155:bool)
          n135 = global read "GlobalMiscellaneous.vi" "Diverting_Power_LimeLight"() -> (w157:bool)
          n136 = global read "GlobalDrivebase.vi" "SEN_Drive_Overheat"() -> (w117:bool[])
          n137 = global read "GlobalDrivebase.vi" "SEN_Azimuth_Fault"() -> (w118:bool[])
          n138 = global read "GlobalDrivebase.vi" "SEN_Shifter_Failure"() -> (w116:bool[])
          n139 = global read "GlobalMiscellaneous.vi" "Diverting_Power_LEDS"() -> (w156:bool)
          n140 = global read "GlobalDrivebase.vi" "SEN_Drive_Fault"() -> (w103:bool[])
          n141 = call "ReducedBWSendToNT.vim"("Value In"=w114, "NT Name"="Battery_Critical" ("Name")) -> ()  [unwired: 1 out]
          n142 = call "ReducedBWSendToNT.vim"("Value In"=w115, "NT Name"="Pressure_Vent" ("Name")) -> ()  [unwired: 1 out]
          n143 = call "ReducedBWSendToNT.vim"("Value In"=w111, "NT Name"="Pressure_Leak" ("Name")) -> ()  [unwired: 1 out]
          n144 = global read "GlobalMiscellaneous.vi" "Number_of_Master_Alarms"() -> (w162:i32)
          n145 = global read "GlobalDriverStationData.vi" "Master_Safety_Override"() -> (w158:bool)
          n146 = Index Array(array=w103) -> (element #1=w102:bool, element #2=w101:bool, element #3=w100:bool, element #4=w99:bool)  [unwired: 4 in]
          n147 = Index Array(array=w118) -> (element #1=w125:bool, element #2=w128:bool, element #3=w131:bool, element #4=w134:bool)  [unwired: 4 in]
          n148 = Index Array(array=w117) -> (element #1=w126:bool, element #2=w129:bool, element #3=w132:bool, element #4=w135:bool)  [unwired: 4 in]
          n149 = Index Array(array=w116) -> (element #1=w127:bool, element #2=w130:bool, element #3=w133:bool, element #4=w136:bool)  [unwired: 4 in]
          n150 = global read "GlobalMiscellaneous.vi" "Master_Alarm"() -> (w161:bool)
          n151 = Compound Arithmetic op=OR(w155, w156, w157) -> (w154:bool)
          n152 = call "ReducedBWSendToNT.vim"("Value In"=w154, "NT Name"="Diverting_Power" ("Name")) -> ()  [unwired: 1 out]
          n153 = global read "GlobalArm.vi" "SEN_Arm_Motor_Over_Current"() -> (w104:bool[])
          n154 = global read "GlobalGripper.vi" "SEN_Gripper_Overheat"() -> (w96:bool)
          n155 = global read "GlobalGripper.vi" "SEN_Gripper_Motor_Fault"() -> (w95:bool)
          n156 = call "ReducedBWSendToNT.vim"("Value In"=w161, "NT Name"="Master_Alarm" ("Name")) -> ()  [unwired: 1 out]
          n157 = global read "GlobalMiscellaneous.vi" "Control_Latency_Alarm"() -> (w112:bool)
          n158 = global read "GlobalArm.vi" "SEN_Arm_Motor_Fault"() -> (w106:bool[])
          n159 = To Double Precision Float(number=w162) -> (double precision float=w163:dbl)
          n160 = global read "GlobalMiscellaneous.vi" "SEN_TOF_Failure"() -> (w94:bool)
          n161 = call "ReducedBWSendToNT.vim"("Value In"=w158, "NT Name"="Robot_in_Safety_Override" ("Name")) -> ()  [unwired: 1 out]
          n162 = global read "GlobalMiscellaneous.vi" "SEN_Electrical_Fault"() -> (w113:bool)
          n163 = Build Array(w125, w126, w127, w102) -> (w137:bool[])
          n164 = Build Array(w128, w129, w130, w101) -> (w138:bool[])
          n165 = Build Array(w131, w132, w133, w100) -> (w139:bool[])
          n166 = Build Array(w134, w135, w136, w99) -> (w140:bool[])
          n167 = global read "GlobalMiscellaneous.vi" "SEN_CAN_Bus_Fault"() -> (w110:bool)
          n168 = global read "GlobalArm.vi" "SEN_Arm_Overheat"() -> (w108:bool[])
          n169 = global read "GlobalAutonomous.vi" "Auto_Error"() -> (w151:errorcluster)
          n170 = call "ReducedBWSendToNT.vim"("Value In"=w163, "NT Name"="Number_of_Master_Alarms" ("Name")) -> ()  [unwired: 1 out]
          n171 = global read "GlobalPoseAndTargeting.vi" "IMU_Failure"() -> (w153:bool)
          n172 = global read "GlobalPoseAndTargeting.vi" "Vision_Fault"() -> (w141:bool)
          n173 = Unbundle(w151) -> ("status"=w152:bool)  [unwired: 2 out]
          n174 = call "ReducedBWSendToNT.vim"("Value In"=w95, "NT Name"="Gripper_Motor_Fault") -> ()  [unwired: 1 out]
          n175 = call "ReducedBWSendToNT.vim"("Value In"=w94, "NT Name"="TOF_Failure") -> ()  [unwired: 1 out]
          n176 = call "ReducedBWSendToNT.vim"("Value In"=w104, "NT Name"="Arm_Motor_Over_Current") -> ()  [unwired: 1 out]
          n177 = call "ReducedBWSendToNT.vim"("Value In"=w106, "NT Name"="Arm_Motor_Fault") -> ()  [unwired: 1 out]
          n178 = call "ReducedBWSendToNT.vim"("Value In"=w96, "NT Name"="Gripper_Overheating") -> ()  [unwired: 1 out]
          n179 = call "ReducedBWSendToNT.vim"("Value In"=w108, "NT Name"="Arm_Overheating") -> ()  [unwired: 1 out]
          n180 = call "ReducedBWSendToNT.vim"("Value In"=w137, "NT Name"="Swerve_0_Errors") -> ()  [unwired: 1 out]
          n181 = call "ReducedBWSendToNT.vim"("Value In"=w138, "NT Name"="Swerve_1_Errors") -> ()  [unwired: 1 out]
          n182 = call "ReducedBWSendToNT.vim"("Value In"=w139, "NT Name"="Swerve_2_Errors") -> ()  [unwired: 1 out]
          n183 = call "ReducedBWSendToNT.vim"("Value In"=w140, "NT Name"="Swerve_3_Errors") -> ()  [unwired: 1 out]
          n184 = call "ReducedBWSendToNT.vim"("Value In"=w112, "NT Name"="Control_Latency_Alarm" ("Name")) -> ()  [unwired: 1 out]
          n185 = call "ReducedBWSendToNT.vim"("Value In"=w113, "NT Name"="Electrical_Fault" ("Name")) -> ()  [unwired: 1 out]
          n186 = call "ReducedBWSendToNT.vim"("Value In"=w153, "NT Name"="IMU_Failure" ("Name")) -> ()  [unwired: 1 out]
          n187 = call "ReducedBWSendToNT.vim"("Value In"=w152, "NT Name"="Auto_Error" ("Name")) -> ()  [unwired: 1 out]
          n188 = call "ReducedBWSendToNT.vim"("Value In"=w141, "NT Name"="Vision_Fault" ("Name")) -> ()  [unwired: 1 out]
          n189 = call "ReducedBWSendToNT.vim"("Value In"=w110, "NT Name"="CAN_Bus_Fault" ("Name")) -> ()  [unwired: 1 out]
        }
        frame #2 {
          # "tab specific"
          n190 = case shown="3, 7" w164 {
            frame 0, Default {
              # "no tab open"
            }
            frame 1 {
              # "Auto/Setup tab open"
              n191 = global read "GlobalPoseAndTargeting.vi" "Current_Blue_Calibration"() -> (w167:dbl)
              n192 = global read "GlobalPoseAndTargeting.vi" "Current_Red_Calibration"() -> (w170:dbl)
              n193 = global read "GlobalMiscellaneous.vi" "SEN_TOF_Range (in)"() -> (w166:dbl)
              n194 = call "ReducedBWSendToNT.vim"("Value In"=w167, "NT Name"="Current_Blue_Calibration") -> ()  [unwired: 1 out]
              n195 = call "ReducedBWSendToNT.vim"("Value In"=w166, "NT Name"="TOF_Range") -> ()  [unwired: 1 out]
              n196 = call "ReducedBWSendToNT.vim"("Value In"=w170, "NT Name"="Current_Red_Calibration") -> ()  [unwired: 1 out]
            }
            frame 3, 7 {
              # "Tune or Variables tabs are open"
              n197 = global read "GlobalDrivebase.vi" "SEN_Azimuth_Position_2 (deg)"() -> (w205:dbl)
              n198 = global read "GlobalDrivebase.vi" "SEN_Azimuth_Position_1 (deg)"() -> (w209:dbl)
              n199 = global read "GlobalDrivebase.vi" "SEN_Azimuth_Position_3 (deg)"() -> (w201:dbl)
              n200 = global read "GlobalDrivebase.vi" "SEN_Azimuth_Position_0 (deg)"() -> (w213:dbl)
              n201 = global read "GlobalDrivebase.vi" "SEN_Actual_Shifter_State_2"() -> (w202:T4)
              n202 = global read "GlobalDrivebase.vi" "SEN_Actual_Shifter_State_1"() -> (w206:T4)
              n203 = global read "GlobalDrivebase.vi" "SEN_Actual_Shifter_State_3"() -> (w198:T4)
              n204 = global read "GlobalMiscellaneous.vi" "Swerve_Output_Loop_Time (ms)"() -> (w176:u32)
              n205 = global read "GlobalDrivebase.vi" "SEN_Actual_Shifter_State_0"() -> (w210:T4)
              n206 = global read "GlobalDrivebase.vi" "SEN_Drive_Velocity_2 (ft/s)"() -> (w203:dbl)
              n207 = global read "GlobalDrivebase.vi" "SEN_Drive_Velocity_1 (ft/s)"() -> (w207:dbl)
              n208 = global read "GlobalArm.vi" "SEN_Shoulder_Temp (C)"() -> (w187:u8)
              n209 = global read "GlobalDrivebase.vi" "SEN_Drive_Velocity_3 (ft/s)"() -> (w199:dbl)
              n210 = global read "GlobalDrivebase.vi" "SEN_Drive_Velocity_0 (ft/s)"() -> (w211:dbl)
              n211 = global read "GlobalArm.vi" "SEN_Current_Shoulder_Angle (deg)"() -> (w195:dbl)
              n212 = global read "GlobalArm.vi" "SEN_Elbow_Temp (C)"() -> (w186:u8)
              n213 = global read "GlobalArm.vi" "SEN_Current_Elbow_Angle (deg)"() -> (w194:dbl)
              n214 = global read "GlobalArm.vi" "SEN_Wrist_Temp (C)"() -> (w185:u8)
              n215 = global read "GlobalMiscellaneous.vi" "Control_Loop_Time (ms)"() -> (w197:u32)
              n216 = global read "GlobalDrivebase.vi" "SEN_Drive_Temp_2 (C)"() -> (w204:u8)
              n217 = global read "GlobalArm.vi" "SEN_Current_Wrist_Angle (deg)"() -> (w193:dbl)
              n218 = global read "GlobalDrivebase.vi" "SEN_Drive_Temp_1 (C)"() -> (w208:u8)
              n219 = global read "GlobalDrivebase.vi" "SEN_Drive_Temp_3 (C)"() -> (w200:u8)
              n220 = global read "GlobalDrivebase.vi" "SEN_Drive_Temp_0 (C)"() -> (w212:u8)
              n221 = global read "GlobalMiscellaneous.vi" "Pose_Loop_Time (ms)"() -> (w196:u32)
              n222 = global read "GlobalDrivebase.vi" "OUT_Current_Driver_Profile_Setpoints"() -> (w214:dbl[])
              n223 = global read "GlobalGripper.vi" "SEN_Gripper_Temp (C)"() -> (w173:u8)
              n224 = global read "GlobalArm.vi" "OUT_Arm_Goal_Position (in)"() -> (w191:dbl[])
              n225 = global read "GlobalGripper.vi" "SEN_Gripper_Velocity(RPM)"() -> (w171:dbl)
              n226 = global read "GlobalArm.vi" "SEN_End_Effector_Z"() -> (w179:dbl)
              n227 = global read "GlobalArm.vi" "SEN_End_Effector_X"() -> (w180:dbl)
              n228 = Build Array(w187, w186, w185) -> (w188:u8[])
              n229 = To Double Precision Float(number=w188) -> (double precision float=w184:dbl[])
              n230 = Build Array(w195, w194, w193) -> (w189:dbl[])
              n231 = To Double Precision Float(number=w173) -> (double precision float=w175:dbl)
              n232 = To Double Precision Float(number=w208) -> (double precision float=w226:dbl)
              n233 = To Double Precision Float(number=w206) -> (double precision float=w225:dbl)
              n234 = To Double Precision Float(number=w212) -> (double precision float=w230:dbl)
              n235 = To Double Precision Float(number=w204) -> (double precision float=w222:dbl)
              n236 = To Double Precision Float(number=w200) -> (double precision float=w218:dbl)
              n237 = To Double Precision Float(number=w210) -> (double precision float=w229:dbl)
              n238 = To Double Precision Float(number=w202) -> (double precision float=w221:dbl)
              n239 = To Double Precision Float(number=w198) -> (double precision float=w217:dbl)
              n240 = To Double Precision Float(number=w176) -> (double precision float=w177:dbl)
              n241 = To Double Precision Float(number=w197) -> (double precision float=w234:dbl)
              n242 = To Double Precision Float(number=w196) -> (double precision float=w232:dbl)
              n243 = call "ReducedBWSendToNT.vim"("Value In"=w189, "NT Name"="Arm_Current_Angles" ("name")) -> ()  [unwired: 1 out]
              n244 = call "ReducedBWSendToNT.vim"("Value In"=w184, "NT Name"="Arm_Temperatures") -> ()  [unwired: 1 out]
              n245 = call "ReducedBWSendToNT.vim"("Value In"=w191, "NT Name"="Arm_Gripper_Goal" ("name")) -> ()  [unwired: 1 out]
              n246 = call "ReducedBWSendToNT.vim"("Value In"=w175, "NT Name"="Gripper_Temperature") -> ()  [unwired: 1 out]
              n247 = call "ReducedBWSendToNT.vim"("Value In"=w171, "NT Name"="Gripper_Velocity") -> ()  [unwired: 1 out]
              n248 = call "ReducedBWSendToNT.vim"("Value In"=w179, "NT Name"="End_Effector_Z" ("Name")) -> ()  [unwired: 1 out]
              n249 = call "ReducedBWSendToNT.vim"("Value In"=w180, "NT Name"="End_Effector_X" ("Name")) -> ()  [unwired: 1 out]
              n250 = Build Array(w209, w226, w207, w225) -> (w224:dbl[])
              n251 = Build Array(w213, w230, w211, w229) -> (w228:dbl[])
              n252 = Build Array(w205, w222, w203, w221) -> (w220:dbl[])
              n253 = Build Array(w201, w218, w199, w217) -> (w216:dbl[])
              n254 = call "ReducedBWSendToNT.vim"("Value In"=w177, "NT Name"="Swerve_Output_Loop_Time" ("Name")) -> ()  [unwired: 1 out]
              n255 = call "ReducedBWSendToNT.vim"("Value In"=w214, "NT Name"="Current_Driver_Profile_Setpoints" ("Name")) -> ()  [unwired: 1 out]
              n256 = call "ReducedBWSendToNT.vim"("Value In"=w234, "NT Name"="Control_Loop_Time" ("Name")) -> ()  [unwired: 1 out]
              n257 = call "ReducedBWSendToNT.vim"("Value In"=w232, "NT Name"="Pose_Loop_Time" ("Name")) -> ()  [unwired: 1 out]
              n258 = call "ReducedBWSendToNT.vim"("Value In"=w224, "NT Name"="Swerve_1_Details") -> ()  [unwired: 1 out]
              n259 = call "ReducedBWSendToNT.vim"("Value In"=w228, "NT Name"="Swerve_0_Details") -> ()  [unwired: 1 out]
              n260 = call "ReducedBWSendToNT.vim"("Value In"=w220, "NT Name"="Swerve_2_Details") -> ()  [unwired: 1 out]
              n261 = call "ReducedBWSendToNT.vim"("Value In"=w216, "NT Name"="Swerve_3_Details") -> ()  [unwired: 1 out]
            }
          }
        }
      }
    }
  }
